vi "Test Fixed.vi"(8 "error in (no error)":errorcluster) -> (0 "error out":errorcluster)   [LabVIEW 2020]
uses:
  Source/Protobuf RAW/float/float.lvclass/float.ctl
  Source/Protobuf RAW/fixed32/fixed32.lvclass/fixed32.ctl
  Source/Protobuf RAW/sfixed32/sfixed32.lvclass/sfixed32.ctl
  Source/Protobuf RAW/sfixed64/sfixed64.lvclass/sfixed64.ctl
  Source/Protobuf RAW/double/double.lvclass/double.ctl
  Source/Protobuf RAW/fixed64/fixed64.lvclass/fixed64.ctl
  Source/Protobuf RAW/fixed64/Write Value.vi
  Source/Protobuf RAW/double/Write Value.vi
  Source/Protobuf RAW/sfixed64/Write Value.vi
  Source/Protobuf RAW/sfixed32/Write Value.vi
  Source/Protobuf RAW/fixed32/Write Value.vi
  Source/Protobuf RAW/float/Write Value.vi
  <vilib>/addons/_JKI Toolkits/Caraya/classes/Assert/Assert Equal Value and Type_Variant.vi
  Source/Protobuf RAW/float/float.lvclass
  Source/Protobuf RAW/fixed32/fixed32.lvclass
  Source/Protobuf RAW/sfixed32/sfixed32.lvclass
  Source/Protobuf RAW/double/double.lvclass
  Source/Protobuf RAW/fixed64/fixed64.lvclass
  Source/Protobuf RAW/sfixed64/sfixed64.lvclass
  <vilib>/addons/_JKI Toolkits/Caraya/classes/Test/Test.lvclass
  Source/Protobuf RAW.lvlib
  <vilib>/addons/_JKI Toolkits/Caraya/classes/Assert/Assert.lvclass
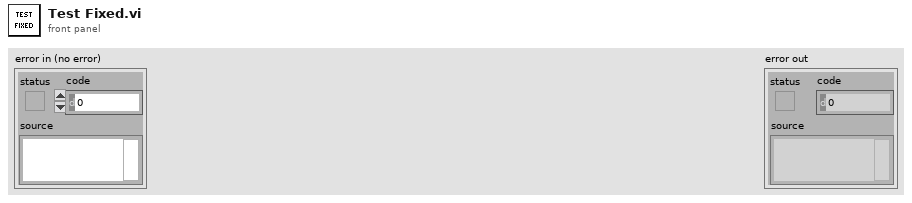
[diagram p1: front panel]
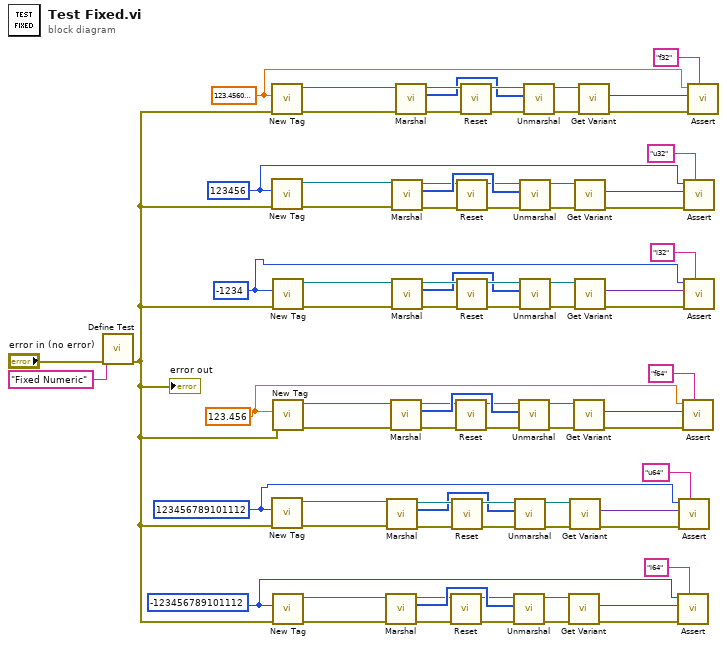
[diagram p0: block diagram]
diagram:
  w2 = i64 -123456789101112 ("Value")
  w3 = u64 123456789101112 ("Value")
  w5 = 123.456 ("Value")
  w4 = -1234 ("Value")
  w56 = u32 123456 ("Value")
  w68 = sgl 123.456 ("Value")
  n1 = call <vilib>:"Define Test.vi"("error in (no error)"="error in (no error)", "Label (VI Title)"="Fixed Numeric") -> ("error out"=w1:errorcluster)  [unwired: 9 in]
  "error out" <- w1
  n2 = call-poly "New Tag.vi"("error in (no error)"=w1, "Value"=w68) -> ("error out"=w79:errorcluster, "float out"=w70:refnum<class "float.lvclass">)  [unwired: 8 in]
  n3 = call-poly "New Tag.vi"("error in (no error)"=w1, "Value"=w56) -> ("error out"=w54:errorcluster, "fixed32 out"=w55:refnum<class "fixed32.lvclass">)  [unwired: 8 in]
  n4 = call-poly "New Tag.vi"("error in (no error)"=w1, "Value"=w3) -> ("error out"=w8:errorcluster, "fixed64 out"=w9:refnum<class "fixed64.lvclass">)  [unwired: 8 in]
  n5 = call-poly "New Tag.vi"("error in (no error)"=w1, "Value"=w4) -> ("error out"=w12:errorcluster, "sfixed32 out"=w13:refnum<class "sfixed32.lvclass">)  [unwired: 8 in]
  n6 = call-poly "New Tag.vi"("error in (no error)"=w1, "Value"=w5) -> ("error out"=w10:errorcluster, "double out"=w11:refnum<class "double.lvclass">)  [unwired: 8 in]
  n7 = call-poly "New Tag.vi"("error in (no error)"=w1, "Value"=w2) -> ("error out"=w6:errorcluster, "sfixed64 out"=w7:refnum<class "sfixed64.lvclass">)  [unwired: 8 in]
  n8 = call-dynamic "Marshal.vi"("error in (no error)"=w6, "int32 in"=w7) -> ("error out"=w15:errorcluster, "Buffer"=w18:u8[], "int32 out"=w14:refnum<class "sfixed64.lvclass">)  [unwired: 7 in]
  n9 = call-dynamic "Marshal.vi"("error in (no error)"=w8, "int32 in"=w9) -> ("error out"=w32:errorcluster, "Buffer"=w29:u8[], "int32 out"=w33:refnum<class "fixed64.lvclass">)  [unwired: 7 in]
  n10 = call-dynamic "Marshal.vi"("error in (no error)"=w10, "int32 in"=w11) -> ("error out"=w35:errorcluster, "Buffer"=w38:u8[], "int32 out"=w34:refnum<class "double.lvclass">)  [unwired: 7 in]
  n11 = call-dynamic "Marshal.vi"("error in (no error)"=w54, "int32 in"=w55) -> ("error out"=w58:errorcluster, "Buffer"=w61:u8[], "int32 out"=w57:refnum<class "fixed32.lvclass">)  [unwired: 7 in]
  n12 = call-dynamic "Marshal.vi"("error in (no error)"=w12, "int32 in"=w13) -> ("error out"=w52:errorcluster, "Buffer"=w49:u8[], "int32 out"=w53:refnum<class "sfixed32.lvclass">)  [unwired: 7 in]
  n13 = call-dynamic "Marshal.vi"("error in (no error)"=w79, "int32 in"=w70) -> ("error out"=w77:errorcluster, "Buffer"=w74:u8[], "int32 out"=w78:refnum<class "float.lvclass">)  [unwired: 7 in]
  n14 = call-dynamic "Reset.vi"("error in (no error)"=w15, "Proto Tag in"=w14) -> ("error out"=w17:errorcluster, "Proto Tag out"=w16:refnum<class "sfixed64.lvclass">)  [unwired: 8 in]
  n15 = call-dynamic "Reset.vi"("error in (no error)"=w32, "Proto Tag in"=w33) -> ("error out"=w30:errorcluster, "Proto Tag out"=w31:refnum<class "fixed64.lvclass">)  [unwired: 8 in]
  n16 = call-dynamic "Reset.vi"("error in (no error)"=w35, "Proto Tag in"=w34) -> ("error out"=w37:errorcluster, "Proto Tag out"=w36:refnum<class "double.lvclass">)  [unwired: 8 in]
  n17 = call-dynamic "Reset.vi"("error in (no error)"=w58, "Proto Tag in"=w57) -> ("error out"=w60:errorcluster, "Proto Tag out"=w59:refnum<class "fixed32.lvclass">)  [unwired: 8 in]
  n18 = call-dynamic "Reset.vi"("error in (no error)"=w52, "Proto Tag in"=w53) -> ("error out"=w50:errorcluster, "Proto Tag out"=w51:refnum<class "sfixed32.lvclass">)  [unwired: 8 in]
  n19 = call-dynamic "Reset.vi"("error in (no error)"=w77, "Proto Tag in"=w78) -> ("error out"=w75:errorcluster, "Proto Tag out"=w76:refnum<class "float.lvclass">)  [unwired: 8 in]
  n20 = call-dynamic "Unmarshal.vi"("error in (no error)"=w17, "Buffer"=w18, "int32 in"=w16) -> ("error out"=w19:errorcluster, "int32 out"=w20:refnum<class "sfixed64.lvclass">)  [unwired: 6 in, 1 out]
  n21 = call-dynamic "Unmarshal.vi"("error in (no error)"=w30, "Buffer"=w29, "int32 in"=w31) -> ("error out"=w28:errorcluster, "int32 out"=w27:refnum<class "fixed64.lvclass">)  [unwired: 6 in, 1 out]
  n22 = call-dynamic "Unmarshal.vi"("error in (no error)"=w37, "Buffer"=w38, "int32 in"=w36) -> ("error out"=w39:errorcluster, "int32 out"=w40:refnum<class "double.lvclass">)  [unwired: 6 in, 1 out]
  n23 = call-dynamic "Unmarshal.vi"("error in (no error)"=w60, "Buffer"=w61, "int32 in"=w59) -> ("error out"=w62:errorcluster, "int32 out"=w63:refnum<class "fixed32.lvclass">)  [unwired: 6 in, 1 out]
  n24 = call-dynamic "Unmarshal.vi"("error in (no error)"=w50, "Buffer"=w49, "int32 in"=w51) -> ("error out"=w48:errorcluster, "int32 out"=w47:refnum<class "sfixed32.lvclass">)  [unwired: 6 in, 1 out]
  n25 = call-dynamic "Unmarshal.vi"("error in (no error)"=w75, "Buffer"=w74, "int32 in"=w76) -> ("error out"=w73:errorcluster, "int32 out"=w72:refnum<class "float.lvclass">)  [unwired: 6 in, 1 out]
  n26 = call-dynamic "Get Variant.vi"("error in (no error)"=w19, "int32 in"=w20) -> ("error out"=w21:errorcluster, "Variant"=w22:variant)  [unwired: 7 in, 1 out]
  n27 = call-dynamic "Get Variant.vi"("error in (no error)"=w28, "int32 in"=w27) -> ("error out"=w26:errorcluster, "Variant"=w25:variant)  [unwired: 7 in, 1 out]
  n28 = call-dynamic "Get Variant.vi"("error in (no error)"=w39, "int32 in"=w40) -> ("error out"=w41:errorcluster, "Variant"=w42:variant)  [unwired: 7 in, 1 out]
  n29 = call-dynamic "Get Variant.vi"("error in (no error)"=w62, "int32 in"=w63) -> ("error out"=w64:errorcluster, "Variant"=w65:variant)  [unwired: 7 in, 1 out]
  n30 = call-dynamic "Get Variant.vi"("error in (no error)"=w48, "int32 in"=w47) -> ("error out"=w46:errorcluster, "Variant"=w45:variant)  [unwired: 7 in, 1 out]
  n31 = call-dynamic "Get Variant.vi"("error in (no error)"=w73, "int32 in"=w72) -> ("error out"=w71:errorcluster, "Variant"=w69:variant)  [unwired: 7 in, 1 out]
  n32 = call-poly <vilib>:"Assert.vi"("Label"="i64", "error in (no error)"=w21, "Y"=w22, "X"=w2) -> ()  [unwired: 7 in, 1 out]
  n33 = call-poly <vilib>:"Assert.vi"("Label"="u64", "error in (no error)"=w26, "Y"=w25, "X"=w3) -> ()  [unwired: 7 in, 1 out]
  n34 = call-poly <vilib>:"Assert.vi"("Label"="f64", "error in (no error)"=w41, "Y"=w42, "X"=w5) -> ()  [unwired: 7 in, 1 out]
  n35 = call-poly <vilib>:"Assert.vi"("Label"="u32", "error in (no error)"=w64, "Y"=w65, "X"=w56) -> ()  [unwired: 7 in, 1 out]
  n36 = call-poly <vilib>:"Assert.vi"("Label"="i32", "error in (no error)"=w46, "Y"=w45, "X"=w4) -> ()  [unwired: 7 in, 1 out]
  n37 = call-poly <vilib>:"Assert.vi"("Label"="f32", "error in (no error)"=w71, "Y"=w69, "X"=w68) -> ()  [unwired: 7 in, 1 out]
